vi "dB(T)_2024.vi"(14 "Temperature (K)":dbl=373.15 format="%.4g") -> (0 "T^2*d^2Bair/dT^2":dbl=-9.863442284460733e-05 format="%#_6e", 1 "T*dBair/dT":dbl=4.3077522102604444e-05, 3 "T*dBwater/dT":dbl=0.0016857833537860616 format="%#_6e", 4 "T^2*d^2Bwater/dT^2":dbl=-0.009822685834053062 format="%#_6e", 7 "d^2Bair-water/dT^2":dbl=-1.0645256351379218e-09, 8 "T^2*d^2Bair-water/dT^2":dbl=-0.0001482255314615026 format="%_6e", 9 "dBair-water/dT":dbl=1.5861556674262897e-07, 10 "T*dBair-water/dT":dbl=5.9187398730011994e-05, 11 "dBair/dT":dbl=1.1544291063273333e-07, 12 "d^2Bair/dT^2":dbl=-7.083723741101137e-10, 13 "d^2Bwater/dT^2":dbl=-7.054453286930115e-08, 15 "dBwater/dT":dbl=4.517709644341583e-06)   [LabVIEW 2016]
uses:
  SOS_Global_2022.vi
  <vilib>/gmath/NI_Gmath.lvlib
  <vilib>/Analysis/NI_AALPro.lvlib
panel:
  in  "method interpolation 5":i32(ring)=2 items=["nearest", "linear", "spline", "cubic Hermite", "Lagrange"]
  in  "method derivatives 5":u16(ring)=2 items=["2nd Order Central", "4th Order Central", "Forward", "Backward"]
  in  "method interpolation 4":i32(ring)=2 items=["nearest", "linear", "spline", "cubic Hermite", "Lagrange"]
  in  "method derivatives 4":u16(ring)=2 items=["2nd Order Central", "4th Order Central", "Forward", "Backward"]
  in  "method interpolation 3":i32(ring)=2 items=["nearest", "linear", "spline", "cubic Hermite", "Lagrange"]
  in  "method derivatives 3":u16(ring)=2 items=["2nd Order Central", "4th Order Central", "Forward", "Backward"]
  in  "Bdw source air-water interaction virial":i32(listbox)=3
  in  "Bw source ref water":i32(listbox)=2
  in  "method derivatives 2":u16(ring)=2 items=["2nd Order Central", "4th Order Central", "Forward", "Backward"]
  in  "method interpolation 2":i32(ring)=2 items=["nearest", "linear", "spline", "cubic Hermite", "Lagrange"]
  in  "method derivatives":u16(ring)=2 items=["2nd Order Central", "4th Order Central", "Forward", "Backward"]
  in  "method interpolation":i32(ring)=2 items=["nearest", "linear", "spline", "cubic Hermite", "Lagrange"]
  in  "B source ref dry air":i32(listbox)=1
  # "(m^3 mol^-1)"
  # "(m^3 mol^-1 K^-1)"
  # "(m^3 mol^-1 K^-2)"
  # "(m^3 mol^-1)"
  # "(m^3 mol^-1)"
  # "(m^3 mol^-1 K^-1)"
  # "(m^3 mol^-1)"
  # "(m^3 mol^-1 K^-2)"
  # "(m^3 mol^-1)"
  # "(m^3 mol^-1 K^-1)"
  # "(m^3 mol^-1)"
  # "(m^3 mol^-1 K^-2)"
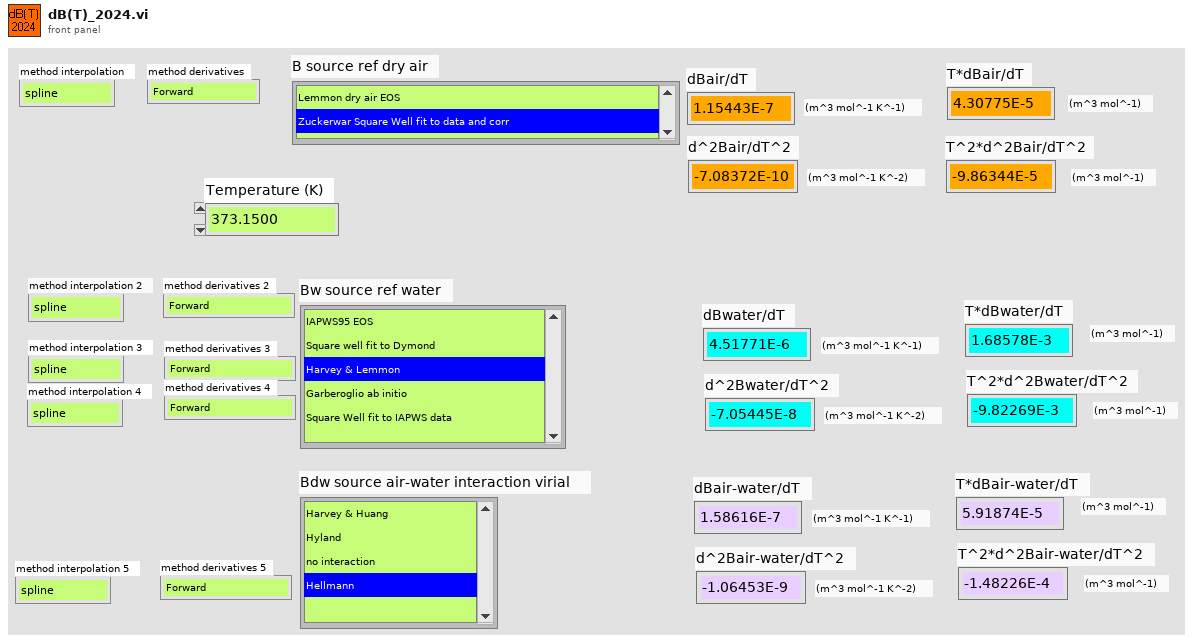
[diagram p1: front panel]
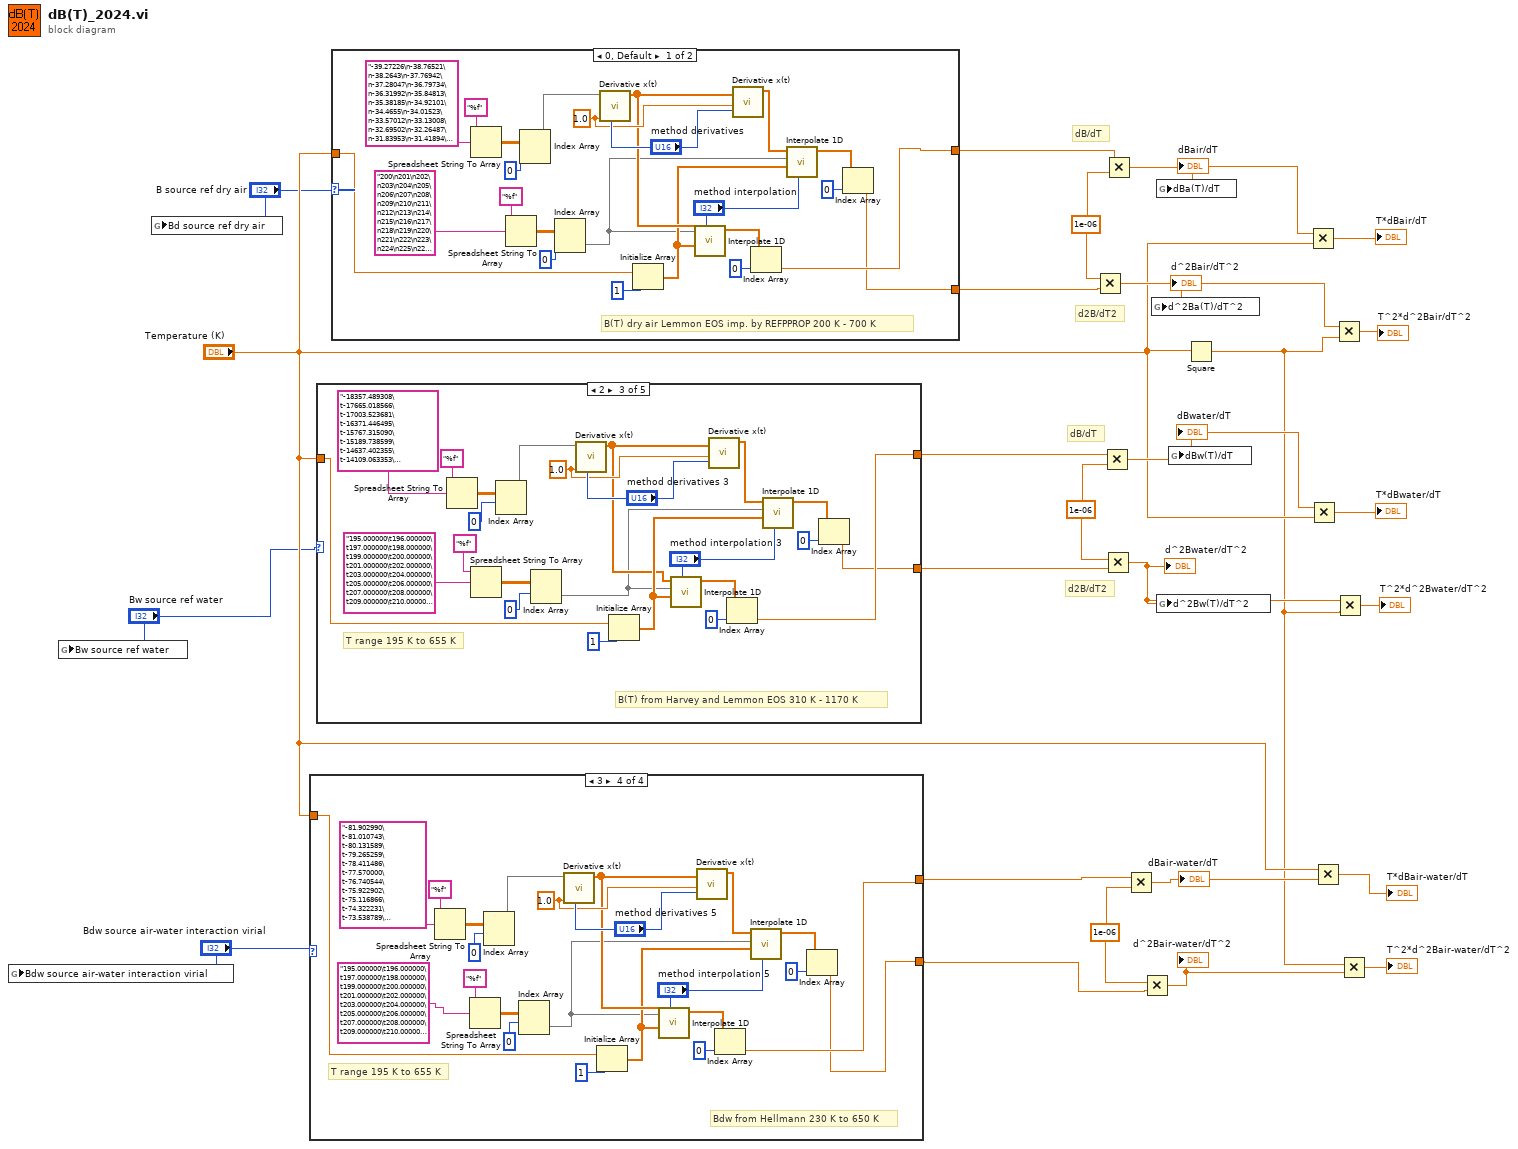
[diagram p0: block diagram]
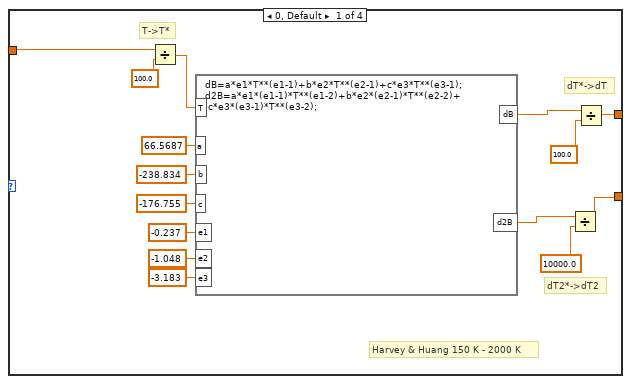
[diagram p2: hidden frame]
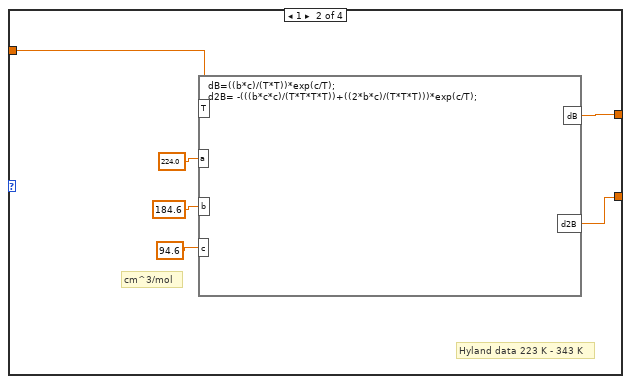
[diagram p3: hidden frame]
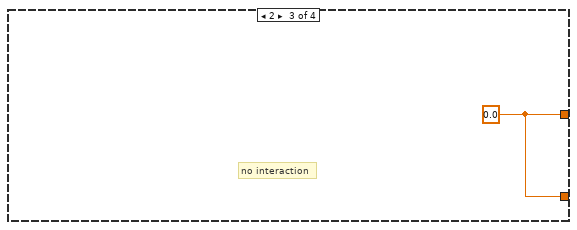
[diagram p4: hidden frame]
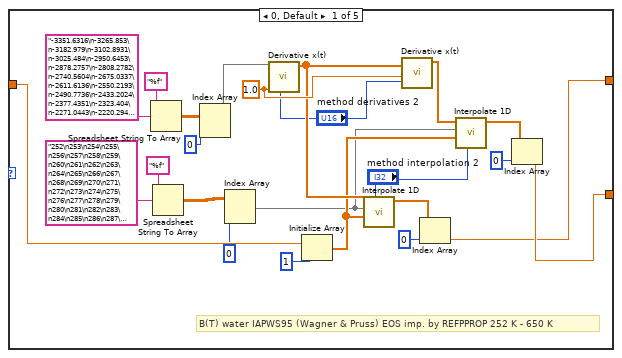
[diagram p5: hidden frame]
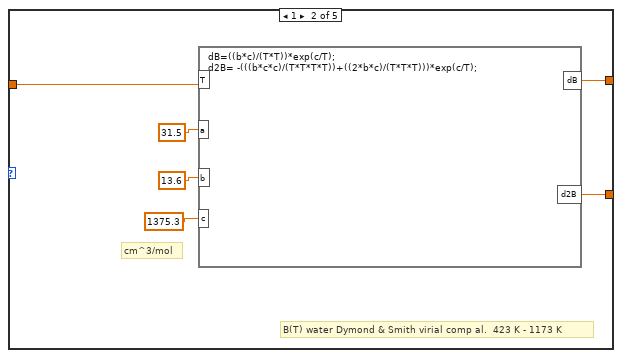
[diagram p6: hidden frame]
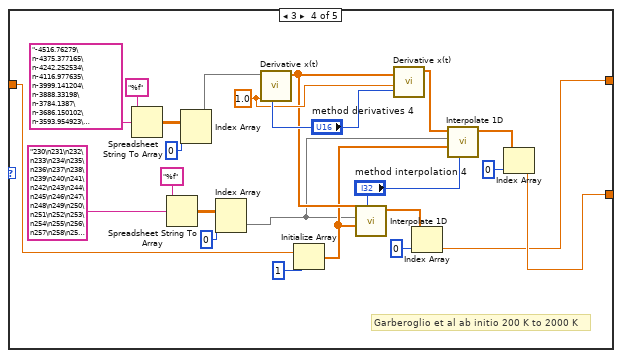
[diagram p7: hidden frame]
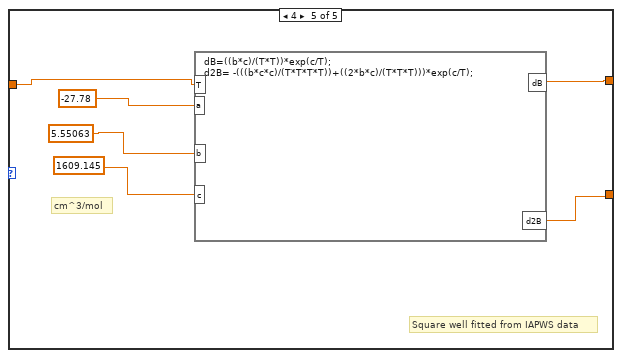
[diagram p8: hidden frame]
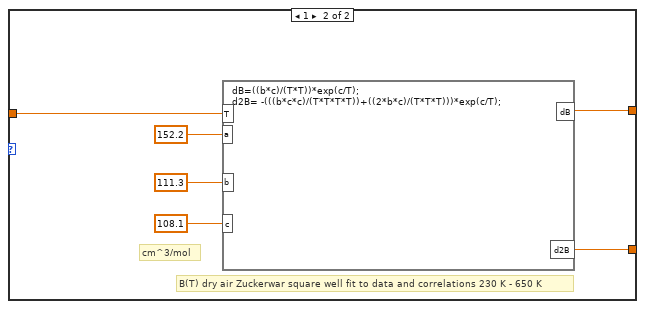
[diagram p9: hidden frame]
diagram:
  w12 = 1e-06 ("y")
  w22 = 1e-06 ("y")
  w23 = 1e-06 ("y")
  # "d2B/dT2"
  # "dB/dT"
  # "d2B/dT2"
  # "dB/dT"
  n1 = global write "SOS_Global_2022.vi" "Bdw source air-water interaction virial"("Bdw source air-water interaction virial") -> ()
  n2 = global write "SOS_Global_2022.vi" "Bw source ref water"("Bw source ref water") -> ()
  n3 = global write "SOS_Global_2022.vi" "Bd source ref dry air"("B source ref dry air") -> ()
  n4 = case shown="3" "Bdw source air-water interaction virial" {
    tunnel: [w31 w44 w48 w55] -> w10
    tunnel: [w30 w43 w48 w54] -> w11
    tunnel: "Temperature (K)" -> [w40 w42 _ w56]
    frame 0, Default {
      # "dT2*->dT2"
      # "dT*->dT"
      # "T->T*"
      # "Harvey & Huang 150 K - 2000 K"
      n5 = Divide(x=w40, y=100.0) -> (x/y=w39:dbl)
      n6 = formula code="dB=a*e1*T**(e1-1)+b*e2*T**(e2-1)+c*e3*T**(e3-1);\nd2B=a*e1*(e1-1)*T**(e1-2)+b*e2*(e2-1)*T**(e2-2)+\n c*e3*(e3-1)*T**(e3-2);"("T"=w39, "a"=66.5687 ("input variable"), "b"=-238.834 ("input variable"), "c"=-176.755 ("input variable"), "e1"=-0.237 ("input variable"), "e2"=-1.048 ("input variable"), "e3"=-3.183 ("input variable")) -> ("dB"=w32:dbl, "d2B"=w28:dbl)
      n7 = Divide(x=w28, y=10000.0) -> (x/y=w30:dbl)
      n8 = Divide(x=w32, y=100.0) -> (x/y=w31:dbl)
    }
    frame 1 {
      # "Hyland data 223 K - 343 K"
      # "cm^3/mol"
      n9 = formula code="dB=((b*c)/(T*T))*exp(c/T);\nd2B= -(((b*c*c)/(T*T*T*T))+((2*b*c)/(T*T*T)))*exp(c/T);"("T"=w42, "a"=224.0 ("input variable"), "b"=184.6 ("input variable"), "c"=94.6 ("input variable")) -> ("dB"=w44:dbl, "d2B"=w43:dbl)
    }
    frame 2 {
      w48 = 0.0
      # "no interaction"
    }
    frame 3 {
      w71 = 1.0 ("dt")
      # "T range 195 K to 655 K"
      # "Bdw from Hellmann 230 K to 650 K"
      n10 = Spreadsheet String To Array(format string="%f", spreadsheet string="-81.902990\t-81.010743\t-80.131589\t-79.265259\t-78.411486\t-77.570000\t-76.740544\t-75.922902\t-75.116866\t-74.322231\t-73.538789\t-72.766335\t-72.004661\t-71.253562\t-70.512830\t-69.782260\t-69.061644\t-68.350777\t-67.649452\t-66.957462\t-66.274601\t-65.600662\t-64.935439\t-64.278725\t-63.630314\t-62.990000\t-62.357591\t-61.732959\t-61.115989\t-60.506569\t-59.904585\t-59.309924\t-58.722471\t-58.142115\t-57.568740\t-57.002235\t-56.442484\t-55.889376\t-55.342796\t-54.802631\t-54.268767\t-53.741092\t-53.219491\t-52.703851\t-52.194058\t-51.690000\t-51.191569\t-50.698684\t-50.211270\t-49.729254\t-49.252559\t-48.781111\t-48.314836\t-47.853660\t-47.397506\t-46.946301\t-46.499970\t-46.058439\t-45.621632\t-45.189475\t-44.761893\t-44.338812\t-43.920157\t-43.505853\t-43.095825\t-42.690000\t-42.288305\t-41.890685\t-41.497087\t-41.107457\t-40.721743\t-40.339892\t-39.961851\t-39.587567\t-39.216988\t-38.850061\t-38.486732\t-38.126949\t-37.770660\t-37.417810\t-37.068348\t-36.722221\t-36.379375\t-36.039758\t-35.703318\t-35.370000\t-35.039755\t-34.712545\t-34.388332\t-34.067080\t-33.748752\t-33.433312\t-33.120725\t-32.810952\t-32.503958\t-32.199707\t-31.898161\t-31.599285\t-31.303041\t-31.009395\t-30.718308\t-30.429745\t-30.143669\t-29.860044\t-29.578833\t-29.300000\t-29.023511\t-28.749343\t-28.477474\t-28.207884\t-27.940552\t-27.675458\t-27.412580\t-27.151897\t-26.893390\t-26.637036\t-26.382815\t-26.130707\t-25.880690\t-25.632744\t-25.386847\t-25.142980\t-24.901120\t-24.661248\t-24.423343\t-24.187383\t-23.953347\t-23.721216\t-23.490968\t-23.262583\t-23.036038\t-22.811315\t-22.588391\t-22.367247\t-22.147860\t-21.930211\t-21.714279\t-21.500042\t-21.287480\t-21.076572\t-20.867297\t-20.659635\t-20.453564\t-20.249064\t-20.046114\t-19.844693\t-19.644780\t-19.446355\t-19.249396\t-19.053883\t-18.859795\t-18.667111\t-18.475811\t-18.285872\t-18.097276\t-17.910000\t-17.724026\t-17.539342\t-17.355939\t-17.173806\t-16.992934\t-16.813313\t-16.634933\t-16.457785\t-16.281858\t-16.107144\t-15.933631\t-15.761311\t-15.590173\t-15.420208\t-15.251406\t-15.083758\t-14.917252\t-14.751881\t-14.587633\t-14.424499\t-14.262470\t-14.101535\t-13.941685\t-13.782909\t-13.625199\t-13.468544\t-13.312935\t-13.158362\t-13.004814\t-12.852283\t-12.700758\t-12.550230\t-12.400689\t-12.252125\t-12.104528\t-11.957889\t-11.812197\t-11.667444\t-11.523618\t-11.380711\t-11.238713\t-11.097613\t-10.957403\t-10.818072\t-10.679610\t-10.542007\t-10.405255\t-10.269343\t-10.134261\t-10.000000\t-9.866550\t-9.733906\t-9.602062\t-9.471012\t-9.340753\t-9.211277\t-9.082580\t-8.954657\t-8.827502\t-8.701110\t-8.575475\t-8.450593\t-8.326458\t-8.203064\t-8.080407\t-7.958481\t-7.837281\t-7.716800\t-7.597036\t-7.477980\t-7.359630\t-7.241978\t-7.125020\t-7.008751\t-6.893165\t-6.778257\t-6.664021\t-6.550452\t-6.437546\t-6.325296\t-6.213697\t-6.102745\t-5.992433\t-5.882756\t-5.773710\t-5.665288\t-5.557485\t-5.450297\t-5.343717\t-5.237741\t-5.132363\t-5.027578\t-4.923380\t-4.819765\t-4.716726\t-4.614259\t-4.512358\t-4.411018\t-4.310234\t-4.210000\t-4.110311\t-4.011164\t-3.912555\t-3.814480\t-3.716936\t-3.619920\t-3.523427\t-3.427455\t-3.331999\t-3.237057\t-3.142625\t-3.048699\t-2.955276\t-2.862353\t-2.769925\t-2.677989\t-2.586542\t-2.495581\t-2.405101\t-2.315099\t-2.225573\t-2.136517\t-2.047929\t-1.959805\t-1.872142\t-1.784936\t-1.698183\t-1.611881\t-1.526025\t-1.440613\t-1.355640\t-1.271103\t-1.186999\t-1.103323\t-1.020073\t-0.937246\t-0.854836\t-0.772842\t-0.691259\t-0.610084\t-0.529314\t-0.448944\t-0.368972\t-0.289394\t-0.210206\t-0.131405\t-0.052988\t0.025050\t0.102711\t0.180000\t0.256919\t0.333470\t0.409656\t0.485478\t0.560938\t0.636038\t0.710780\t0.785165\t0.859196\t0.932874\t1.006201\t1.079178\t1.151809\t1.224094\t1.296036\t1.367635\t1.438895\t1.509817\t1.580403\t1.650654\t1.720572\t1.790160\t1.859419\t1.928351\t1.996958\t2.065241\t2.133203\t2.200845\t2.268169\t2.335177\t2.401871\t2.468253\t2.534324\t2.600086\t2.665542\t2.730693\t2.795540\t2.860086\t2.924333\t2.988282\t3.051935\t3.115294\t3.178361\t3.241138\t3.303626\t3.365828\t3.427744\t3.489378\t3.550731\t3.611804\t3.672600\t3.733121\t3.793367\t3.853342\t3.913047\t3.972483\t4.031653\t4.090558\t4.149201\t4.207583\t4.265705\t4.323571\t4.381181\t4.438537\t4.495642\t4.552497\t4.609104\t4.665464\t4.721581\t4.777454\t4.833087\t4.888481\t4.943638\t4.998560\t5.053249\t5.107706\t5.161933\t5.215933\t5.269707\t5.323256\t5.376583\t5.429690\t5.482578\t5.535249\t5.587705\t5.639948\t5.691980\t5.743802\t5.795417\t5.846825\t5.898030\t5.949033\t5.999836\t6.050440\t6.100847\t6.151060\t6.201080\t6.250908\t6.300548\t6.350000\t6.399266\t6.448348\t6.497244\t6.545957\t6.594487\t6.642834\t6.690999\t6.738983\t6.786786\t6.834408\t6.881851\t6.929114\t6.976199\t7.023106\t7.069836\t7.116389\t7.162765\t7.208966\t7.254992\t7.300844\t7.346521\t7.392025\t7.437357\t7.482516\t7.527504\t7.572321\t7.616968\t7.661445\t7.705752\t7.749891\t7.793862\t7.837665\t7.881302\t7.924772\t7.968077\t8.011217\t8.054192\t8.097003\t8.139650\t8.182135\t8.224458\t8.266619\t8.308619\t8.350459\t8.392139\t8.433660\t8.475021\t8.516225\t8.557272\t8.598161\t8.638894\t8.679471\t8.719894\t8.760161\t8.800275" ("B dw Hellmann array")) -> (array=w58:dbl[][])  [unwired: 2 in]
      n11 = Spreadsheet String To Array(format string="%f", spreadsheet string="195.000000\t196.000000\t197.000000\t198.000000\t199.000000\t200.000000\t201.000000\t202.000000\t203.000000\t204.000000\t205.000000\t206.000000\t207.000000\t208.000000\t209.000000\t210.000000\t211.000000\t212.000000\t213.000000\t214.000000\t215.000000\t216.000000\t217.000000\t218.000000\t219.000000\t220.000000\t221.000000\t222.000000\t223.000000\t224.000000\t225.000000\t226.000000\t227.000000\t228.000000\t229.000000\t230.000000\t231.000000\t232.000000\t233.000000\t234.000000\t235.000000\t236.000000\t237.000000\t238.000000\t239.000000\t240.000000\t241.000000\t242.000000\t243.000000\t244.000000\t245.000000\t246.000000\t247.000000\t248.000000\t249.000000\t250.000000\t251.000000\t252.000000\t253.000000\t254.000000\t255.000000\t256.000000\t257.000000\t258.000000\t259.000000\t260.000000\t261.000000\t262.000000\t263.000000\t264.000000\t265.000000\t266.000000\t267.000000\t268.000000\t269.000000\t270.000000\t271.000000\t272.000000\t273.000000\t274.000000\t275.000000\t276.000000\t277.000000\t278.000000\t279.000000\t280.000000\t281.000000\t282.000000\t283.000000\t284.000000\t285.000000\t286.000000\t287.000000\t288.000000\t289.000000\t290.000000\t291.000000\t292.000000\t293.000000\t294.000000\t295.000000\t296.000000\t297.000000\t298.000000\t299.000000\t300.000000\t301.000000\t302.000000\t303.000000\t304.000000\t305.000000\t306.000000\t307.000000\t308.000000\t309.000000\t310.000000\t311.000000\t312.000000\t313.000000\t314.000000\t315.000000\t316.000000\t317.000000\t318.000000\t319.000000\t320.000000\t321.000000\t322.000000\t323.000000\t324.000000\t325.000000\t326.000000\t327.000000\t328.000000\t329.000000\t330.000000\t331.000000\t332.000000\t333.000000\t334.000000\t335.000000\t336.000000\t337.000000\t338.000000\t339.000000\t340.000000\t341.000000\t342.000000\t343.000000\t344.000000\t345.000000\t346.000000\t347.000000\t348.000000\t349.000000\t350.000000\t351.000000\t352.000000\t353.000000\t354.000000\t355.000000\t356.000000\t357.000000\t358.000000\t359.000000\t360.000000\t361.000000\t362.000000\t363.000000\t364.000000\t365.000000\t366.000000\t367.000000\t368.000000\t369.000000\t370.000000\t371.000000\t372.000000\t373.000000\t374.000000\t375.000000\t376.000000\t377.000000\t378.000000\t379.000000\t380.000000\t381.000000\t382.000000\t383.000000\t384.000000\t385.000000\t386.000000\t387.000000\t388.000000\t389.000000\t390.000000\t391.000000\t392.000000\t393.000000\t394.000000\t395.000000\t396.000000\t397.000000\t398.000000\t399.000000\t400.000000\t401.000000\t402.000000\t403.000000\t404.000000\t405.000000\t406.000000\t407.000000\t408.000000\t409.000000\t410.000000\t411.000000\t412.000000\t413.000000\t414.000000\t415.000000\t416.000000\t417.000000\t418.000000\t419.000000\t420.000000\t421.000000\t422.000000\t423.000000\t424.000000\t425.000000\t426.000000\t427.000000\t428.000000\t429.000000\t430.000000\t431.000000\t432.000000\t433.000000\t434.000000\t435.000000\t436.000000\t437.000000\t438.000000\t439.000000\t440.000000\t441.000000\t442.000000\t443.000000\t444.000000\t445.000000\t446.000000\t447.000000\t448.000000\t449.000000\t450.000000\t451.000000\t452.000000\t453.000000\t454.000000\t455.000000\t456.000000\t457.000000\t458.000000\t459.000000\t460.000000\t461.000000\t462.000000\t463.000000\t464.000000\t465.000000\t466.000000\t467.000000\t468.000000\t469.000000\t470.000000\t471.000000\t472.000000\t473.000000\t474.000000\t475.000000\t476.000000\t477.000000\t478.000000\t479.000000\t480.000000\t481.000000\t482.000000\t483.000000\t484.000000\t485.000000\t486.000000\t487.000000\t488.000000\t489.000000\t490.000000\t491.000000\t492.000000\t493.000000\t494.000000\t495.000000\t496.000000\t497.000000\t498.000000\t499.000000\t500.000000\t501.000000\t502.000000\t503.000000\t504.000000\t505.000000\t506.000000\t507.000000\t508.000000\t509.000000\t510.000000\t511.000000\t512.000000\t513.000000\t514.000000\t515.000000\t516.000000\t517.000000\t518.000000\t519.000000\t520.000000\t521.000000\t522.000000\t523.000000\t524.000000\t525.000000\t526.000000\t527.000000\t528.000000\t529.000000\t530.000000\t531.000000\t532.000000\t533.000000\t534.000000\t535.000000\t536.000000\t537.000000\t538.000000\t539.000000\t540.000000\t541.000000\t542.000000\t543.000000\t544.000000\t545.000000\t546.000000\t547.000000\t548.000000\t549.000000\t550.000000\t551.000000\t552.000000\t553.000000\t554.000000\t555.000000\t556.000000\t557.000000\t558.000000\t559.000000\t560.000000\t561.000000\t562.000000\t563.000000\t564.000000\t565.000000\t566.000000\t567.000000\t568.000000\t569.000000\t570.000000\t571.000000\t572.000000\t573.000000\t574.000000\t575.000000\t576.000000\t577.000000\t578.000000\t579.000000\t580.000000\t581.000000\t582.000000\t583.000000\t584.000000\t585.000000\t586.000000\t587.000000\t588.000000\t589.000000\t590.000000\t591.000000\t592.000000\t593.000000\t594.000000\t595.000000\t596.000000\t597.000000\t598.000000\t599.000000\t600.000000\t601.000000\t602.000000\t603.000000\t604.000000\t605.000000\t606.000000\t607.000000\t608.000000\t609.000000\t610.000000\t611.000000\t612.000000\t613.000000\t614.000000\t615.000000\t616.000000\t617.000000\t618.000000\t619.000000\t620.000000\t621.000000\t622.000000\t623.000000\t624.000000\t625.000000\t626.000000\t627.000000\t628.000000\t629.000000\t630.000000\t631.000000\t632.000000\t633.000000\t634.000000\t635.000000\t636.000000\t637.000000\t638.000000\t639.000000\t640.000000\t641.000000\t642.000000\t643.000000\t644.000000\t645.000000\t646.000000\t647.000000\t648.000000\t649.000000\t650.000000\t651.000000\t652.000000\t653.000000\t654.000000\t655.000000" ("string T array")) -> (array=w60:dbl[][])  [unwired: 2 in]
      n12 = Index Array(array=w58, index (row)=0 ("disabled index (col)")) -> (element=w57:dbl[])  [unwired: 1 in]
      n13 = Index Array(array=w60, index (row)=0 ("disabled index (col)")) -> (element=w53:dbl[])  [unwired: 1 in]
      n14 = call <vilib>:"Derivative x(t).vi"("method"="method derivatives 5", "dt"=w71, "X"=w57) -> ("dX/dt"=w64:dbl[])  [unwired: 7 in, 1 out]
      n15 = Initialize Array(w56, 1 ("dimension size")) -> (w63:dbl[])
      n16 = call <vilib>:"Interpolate 1D.vi"("method"="method interpolation 5", "xi"=w63, "X"=w53, "Y"=w64) -> ("yi"=w69:dbl[])  [unwired: 5 in, 2 out]
      n17 = call <vilib>:"Derivative x(t).vi"("method"="method derivatives 5", "dt"=w71, "X"=w64) -> ("dX/dt"=w65:dbl[])  [unwired: 7 in, 1 out]
      n18 = Index Array(array=w69, index=0) -> (element=w55:dbl)
      n19 = call <vilib>:"Interpolate 1D.vi"("method"="method interpolation 5", "xi"=w63, "X"=w53, "Y"=w65) -> ("yi"=w67:dbl[])  [unwired: 5 in, 2 out]
      n20 = Index Array(array=w67, index=0) -> (element=w54:dbl)
    }
  }
  n21 = case shown="2" "Bw source ref water" {
    tunnel: [w85 w99 w111 w129 w153] -> w25
    tunnel: [w86 w98 w110 w130 w152] -> w21
    tunnel: "Temperature (K)" -> [w83 w97 w112 w131 w151]
    frame 0, Default {
      w96 = 1.0 ("dt")
      # "B(T) water IAPWS95 (Wagner & Pruss) EOS imp. by REFPPROP 252 K - 650 K"
      n22 = Spreadsheet String To Array(format string="%f", spreadsheet string="-3351.6316\n-3265.853\n-3182.979\n-3102.8931\n-3025.484\n-2950.6453\n-2878.2757\n-2808.2782\n-2740.5604\n-2675.0337\n-2611.6136\n-2550.2193\n-2490.7736\n-2433.2024\n-2377.4351\n-2323.404\n-2271.0443\n-2220.294\n-2171.0936\n-2123.3865\n-2077.1179\n-2032.2357\n-1988.6898\n-1946.4323\n-1905.4172\n-1865.6002\n-1826.9391\n-1789.3932\n-1752.9236\n-1717.4929\n-1683.065\n-1649.6055\n-1617.0813\n-1585.4606\n-1554.7126\n-1524.8081\n-1495.7188\n-1467.4174\n-1439.8779\n-1413.0752\n-1386.985\n-1361.5841\n-1336.8502\n-1312.7616\n-1289.2976\n-1266.4383\n-1244.1643\n-1222.4573\n-1201.2993\n-1180.6731\n-1160.5622\n-1140.9505\n-1121.8228\n-1103.164\n-1084.96\n-1067.1968\n-1049.8612\n-1032.9402\n-1016.4216\n-1000.2932\n-984.54359\n-969.16154\n-954.13627\n-939.45738\n-925.1148\n-911.09882\n-897.40004\n-884.0094\n-870.91812\n-858.11771\n-845.59999\n-833.35702\n-821.38114\n-809.66492\n-798.2012\n-786.98303\n-776.0037\n-765.25669\n-754.73573\n-744.43471\n-734.34773\n-724.46907\n-714.79322\n-705.3148\n-696.02862\n-686.92965\n-678.01302\n-669.27399\n-660.70798\n-652.31057\n-644.07743\n-636.00439\n-628.08741\n-620.32255\n-612.706\n-605.23407\n-597.90317\n-590.70981\n-583.65063\n-576.72233\n-569.92173\n-563.24575\n-556.69137\n-550.25568\n-543.93585\n-537.72913\n-531.63285\n-525.6444\n-519.76126\n-513.98098\n-508.30118\n-502.71953\n-497.23378\n-491.84174\n-486.54128\n-481.33032\n-476.20686\n-471.16892\n-466.2146\n-461.34205\n-456.54945\n-451.83504\n-447.19713\n-442.63403\n-438.14413\n-433.72584\n-429.37763\n-425.09801\n-420.8855\n-416.7387\n-412.65621\n-408.63669\n-404.67882\n-400.78132\n-396.94294\n-393.16247\n-389.43872\n-385.77053\n-382.15678\n-378.59636\n-375.08821\n-371.63127\n-368.22453\n-364.86699\n-361.55769\n-358.29567\n-355.08\n-351.9098\n-348.78417\n-345.70225\n-342.66322\n-339.66625\n-336.71053\n-333.7953\n-330.91978\n-328.08323\n-325.28492\n-322.52415\n-319.80022\n-317.11245\n-314.46018\n-311.84275\n-309.25955\n-306.70994\n-304.19333\n-301.70912\n-299.25674\n-296.83561\n-294.4452\n-292.08495\n-289.75434\n-287.45285\n-285.17998\n-282.93524\n-280.71813\n-278.52818\n-276.36494\n-274.22795\n-272.11676\n-270.03094\n-267.97007\n-265.93373\n-263.92151\n-261.93301\n-259.96785\n-258.02564\n-256.106\n-254.20858\n-252.333\n-250.47892\n-248.646\n-246.8339\n-245.04228\n-243.27082\n-241.5192\n-239.78712\n-238.07426\n-236.38033\n-234.70504\n-233.04809\n-231.40921\n-229.78812\n-228.18454\n-226.59822\n-225.02889\n-223.4763\n-221.94019\n-220.42032\n-218.91645\n-217.42834\n-215.95576\n-214.49849\n-213.05629\n-211.62895\n-210.21626\n-208.81799\n-207.43396\n-206.06394\n-204.70775\n-203.36518\n-202.03604\n-200.72015\n-199.41732\n-198.12736\n-196.8501\n-195.58536\n-194.33297\n-193.09275\n-191.86455\n-190.64819\n-189.44352\n-188.25038\n-187.06861\n-185.89806\n-184.73858\n-183.59003\n-182.45225\n-181.3251\n-180.20846\n-179.10217\n-178.0061\n-176.92012\n-175.8441\n-174.77791\n-173.72142\n-172.67451\n-171.63706\n-170.60894\n-169.59004\n-168.58024\n-167.57943\n-166.58749\n-165.60432\n-164.6298\n-163.66382\n-162.70629\n-161.75709\n-160.81613\n-159.88331\n-158.95852\n-158.04167\n-157.13265\n-156.23139\n-155.33778\n-154.45174\n-153.57316\n-152.70198\n-151.83808\n-150.9814\n-150.13185\n-149.28933\n-148.45378\n-147.62511\n-146.80324\n-145.98809\n-145.17958\n-144.37764\n-143.58219\n-142.79316\n-142.01048\n-141.23407\n-140.46386\n-139.69979\n-138.94179\n-138.18978\n-137.4437\n-136.70348\n-135.96907\n-135.24039\n-134.51739\n-133.79999\n-133.08815\n-132.3818\n-131.68087\n-130.98532\n-130.29508\n-129.6101\n-128.93032\n-128.25568\n-127.58614\n-126.92163\n-126.2621\n-125.6075\n-124.95779\n-124.3129\n-123.67279\n-123.03741\n-122.4067\n-121.78063\n-121.15914\n-120.54219\n-119.92972\n-119.3217\n-118.71808\n-118.11881\n-117.52386\n-116.93317\n-116.3467\n-115.76441\n-115.18627\n-114.61222\n-114.04223\n-113.47625\n-112.91426\n-112.3562\n-111.80204\n-111.25175\n-110.70528\n-110.16259\n-109.62366\n-109.08844\n-108.5569\n-108.029\n-107.50471\n-106.98399\n-106.46682\n-105.95314\n-105.44294\n-104.93618\n-104.43283\n-103.93285\n-103.43622\n-102.9429\n-102.45286\n-101.96607\n-101.4825\n-101.00212\n-100.5249\n-100.05082\n-99.57984\n-99.11194\n-98.64708\n-98.18524\n-97.72639\n-97.27052\n-96.81757\n-96.36755\n-95.9204\n-95.47612\n-95.03467\n-94.59603\n-94.16017\n-93.72708\n-93.29672\n-92.86907\n-92.44411\n-92.02181\n-91.60216\n-91.18512\n-90.77067\n-90.3588\n-89.94948\n-89.54269\n-89.1384\n-88.73659\n-88.33726\n-87.94036\n-87.54588\n-87.15381\n-86.76412\n-86.37678\n-85.99179\n-85.60912\n-85.22875\n-84.85067\n-84.47484\n-84.10126\n-83.72991\n-83.36076\n-82.9938\n-82.62901\n-82.26638\n-81.90588\n-81.5475\n-81.19122\n-80.83702\n-80.48489\n-80.13481\n-79.78676") -> (array=w78:dbl[][])  [unwired: 2 in]
      n23 = Spreadsheet String To Array(format string="%f", spreadsheet string="252\n253\n254\n255\n256\n257\n258\n259\n260\n261\n262\n263\n264\n265\n266\n267\n268\n269\n270\n271\n272\n273\n274\n275\n276\n277\n278\n279\n280\n281\n282\n283\n284\n285\n286\n287\n288\n289\n290\n291\n292\n293\n294\n295\n296\n297\n298\n299\n300\n301\n302\n303\n304\n305\n306\n307\n308\n309\n310\n311\n312\n313\n314\n315\n316\n317\n318\n319\n320\n321\n322\n323\n324\n325\n326\n327\n328\n329\n330\n331\n332\n333\n334\n335\n336\n337\n338\n339\n340\n341\n342\n343\n344\n345\n346\n347\n348\n349\n350\n351\n352\n353\n354\n355\n356\n357\n358\n359\n360\n361\n362\n363\n364\n365\n366\n367\n368\n369\n370\n371\n372\n373\n374\n375\n376\n377\n378\n379\n380\n381\n382\n383\n384\n385\n386\n387\n388\n389\n390\n391\n392\n393\n394\n395\n396\n397\n398\n399\n400\n401\n...") -> (array=w81:dbl[][])  [unwired: 2 in]
      n24 = Index Array(array=w78, index (col)=0 ("disabled index (col)")) -> (element=w74:dbl[])  [unwired: 1 in]
      n25 = Index Array(array=w81, index (col)=0 ("disabled index (col)")) -> (element=w73:dbl[])  [unwired: 1 in]
      n26 = call <vilib>:"Derivative x(t).vi"("method"="method derivatives 2", "dt"=w96, "X"=w74) -> ("dX/dt"=w89:dbl[])  [unwired: 7 in, 1 out]
      n27 = Initialize Array(w83, 1 ("dimension size")) -> (w88:dbl[])
      n28 = call <vilib>:"Interpolate 1D.vi"("method"="method interpolation 2", "xi"=w88, "X"=w73, "Y"=w89) -> ("yi"=w94:dbl[])  [unwired: 5 in, 2 out]
      n29 = call <vilib>:"Derivative x(t).vi"("method"="method derivatives 2", "dt"=w96, "X"=w89) -> ("dX/dt"=w90:dbl[])  [unwired: 7 in, 1 out]
      n30 = Index Array(array=w94, index=0) -> (element=w85:dbl)
      n31 = call <vilib>:"Interpolate 1D.vi"("method"="method interpolation 2", "xi"=w88, "X"=w73, "Y"=w90) -> ("yi"=w92:dbl[])  [unwired: 5 in, 2 out]
      n32 = Index Array(array=w92, index=0) -> (element=w86:dbl)
    }
    frame 1 {
      # "B(T) water Dymond & Smith virial comp al.  423 K - 1173 K"
      # "cm^3/mol"
      n33 = formula code="dB=((b*c)/(T*T))*exp(c/T);\nd2B= -(((b*c*c)/(T*T*T*T))+((2*b*c)/(T*T*T)))*exp(c/T);"("T"=w97, "a"=31.5 ("input variable"), "b"=13.6 ("input variable"), "c"=1375.3 ("input variable")) -> ("dB"=w99:dbl, "d2B"=w98:dbl)
    }
    frame 2 {
      w125 = 1.0 ("dt")
      # "T range 195 K to 655 K"
      # "B(T) from Harvey and Lemmon EOS 310 K - 1170 K"
      n34 = Spreadsheet String To Array(format string="%f", spreadsheet string="-18357.489308\t-17665.018566\t-17003.523681\t-16371.446495\t-15767.315090\t-15189.738599\t-14637.402355\t-14109.063353\t-13603.546005\t-13119.738158\t-12656.587379\t-12213.097459\t-11788.325153\t-11381.377113\t-10991.407015\t-10617.612868\t-10259.234487\t-9915.551116\t-9585.879208\t-9269.570329\t-8966.009198\t-8674.611835\t-8394.823834\t-8126.118725\t-7867.996445\t-7619.981892\t-7381.623567\t-7152.492297\t-6932.180032\t-6720.298710\t-6516.479192\t-6320.370249\t-6131.637624\t-5949.963127\t-5775.043802\t-5606.591122\t-5444.330246\t-5287.999305\t-5137.348738\t-4992.140656\t-4852.148249\t-4717.155220\t-4586.955255\t-4461.351516\t-4340.156169\t-4223.189931\t-4110.281646\t-4001.267879\t-3895.992540\t-3794.306519\t-3696.067345\t-3601.138863\t-3509.390928\t-3420.699114\t-3334.944438\t-3252.013100\t-3171.796234\t-3094.189677\t-3019.093744\t-2946.413014\t-2876.056137\t-2807.935638\t-2741.967737\t-2678.072179\t-2616.172074\t-2556.193734\t-2498.066536\t-2441.722776\t-2387.097538\t-2334.128567\t-2282.756150\t-2232.923004\t-2184.574163\t-2137.656875\t-2092.120510\t-2047.916459\t-2004.998048\t-1963.320453\t-1922.840620\t-1883.517186\t-1845.310409\t-1808.182094\t-1772.095528\t-1737.015420\t-1702.907834\t-1669.740137\t-1637.480939\t-1606.100048\t-1575.568409\t-1545.858066\t-1516.942111\t-1488.794643\t-1461.390724\t-1434.706342\t-1408.718370\t-1383.404533\t-1358.743371\t-1334.714205\t-1311.297109\t-1288.472878\t-1266.222998\t-1244.529617\t-1223.375525\t-1202.744121\t-1182.619393\t-1162.985895\t-1143.828722\t-1125.133492\t-1106.886324\t-1089.073819\t-1071.683041\t-1054.701499\t-1038.117131\t-1021.918286\t-1006.093710\t-990.632529\t-975.524239\t-960.758685\t-946.326053\t-932.216857\t-918.421926\t-904.932389\t-891.739672\t-878.835477\t-866.211781\t-853.860819\t-841.775079\t-829.947291\t-818.370418\t-807.037649\t-795.942389\t-785.078253\t-774.439057\t-764.018813\t-753.811719\t-743.812156\t-734.014677\t-724.414007\t-715.005031\t-705.782793\t-696.742486\t-687.879453\t-679.189176\t-670.667273\t-662.309496\t-654.111722\t-646.069953\t-638.180309\t-630.439025\t-622.842447\t-615.387028\t-608.069325\t-600.885996\t-593.833795\t-586.909569\t-580.110259\t-573.432890\t-566.874573\t-560.432503\t-554.103952\t-547.886270\t-541.776881\t-535.773283\t-529.873040\t-524.073786\t-518.373221\t-512.769106\t-507.259266\t-501.841583\t-496.513997\t-491.274506\t-486.121160\t-481.052060\t-476.065361\t-471.159265\t-466.332023\t-461.581931\t-456.907330\t-452.306605\t-447.778183\t-443.320532\t-438.932159\t-434.611611\t-430.357470\t-426.168357\t-422.042925\t-417.979864\t-413.977896\t-410.035774\t-406.152284\t-402.326242\t-398.556492\t-394.841909\t-391.181393\t-387.573874\t-384.018305\t-380.513667\t-377.058965\t-373.653227\t-370.295505\t-366.984875\t-363.720433\t-360.501299\t-357.326610\t-354.195527\t-351.107230\t-348.060916\t-345.055803\t-342.091126\t-339.166139\t-336.280111\t-333.432330\t-330.622098\t-327.848735\t-325.111575\t-322.409968\t-319.743277\t-317.110882\t-314.512174\t-311.946559\t-309.413456\t-306.912296\t-304.442524\t-302.003595\t-299.594978\t-297.216152\t-294.866608\t-292.545848\t-290.253384\t-287.988739\t-285.751446\t-283.541048\t-281.357096\t-279.199154\t-277.066792\t-274.959589\t-272.877135\t-270.819026\t-268.784869\t-266.774276\t-264.786869\t-262.822277\t-260.880137\t-258.960093\t-257.061795\t-255.184901\t-253.329078\t-251.493995\t-249.679332\t-247.884772\t-246.110007\t-244.354732\t-242.618650\t-240.901471\t-239.202906\t-237.522677\t-235.860508\t-234.216128\t-232.589274\t-230.979685\t-229.387107\t-227.811289\t-226.251986\t-224.708957\t-223.181967\t-221.670782\t-220.175176\t-218.694925\t-217.229809\t-215.779614\t-214.344127\t-212.923141\t-211.516452\t-210.123860\t-208.745168\t-207.380184\t-206.028717\t-204.690581\t-203.365593\t-202.053573\t-200.754345\t-199.467734\t-198.193571\t-196.931687\t-195.681919\t-194.444103\t-193.218081\t-192.003697\t-190.800796\t-189.609227\t-188.428843\t-187.259496\t-186.101043\t-184.953343\t-183.816257\t-182.689648\t-181.573382\t-180.467327\t-179.371352\t-178.285331\t-177.209136\t-176.142645\t-175.085735\t-174.038287\t-173.000184\t-171.971308\t-170.951546\t-169.940786\t-168.938916\t-167.945829\t-166.961417\t-165.985575\t-165.018199\t-164.059187\t-163.108438\t-162.165853\t-161.231335\t-160.304788\t-159.386117\t-158.475229\t-157.572033\t-156.676438\t-155.788356\t-154.907698\t-154.034378\t-153.168312\t-152.309416\t-151.457607\t-150.612804\t-149.774927\t-148.943897\t-148.119637\t-147.302069\t-146.491118\t-145.686710\t-144.888772\t-144.097231\t-143.312016\t-142.533057\t-141.760284\t-140.993630\t-140.233027\t-139.478409\t-138.729711\t-137.986867\t-137.249815\t-136.518492\t-135.792836\t-135.072786\t-134.358281\t-133.649264\t-132.945675\t-132.247456\t-131.554551\t-130.866903\t-130.184458\t-129.507161\t-128.834957\t-128.167794\t-127.505620\t-126.848381\t-126.196029\t-125.548511\t-124.905779\t-124.267784\t-123.634476\t-123.005809\t-122.381735\t-121.762207\t-121.147180\t-120.536609\t-119.930448\t-119.328654\t-118.731183\t-118.137991\t-117.549037\t-116.964278\t-116.383674\t-115.807183\t-115.234764\t-114.666378\t-114.101986\t-113.541549\t-112.985027\t-112.432385\t-111.883583\t-111.338585\t-110.797355\t-110.259856\t-109.726052\t-109.195910\t-108.669393\t-108.146467\t-107.627099\t-107.111255\t-106.598902\t-106.090008\t-105.584539\t-105.082464\t-104.583751\t-104.088370\t-103.596289\t-103.107478\t-102.621907\t-102.139546\t-101.660365\t-101.184337\t-100.711431\t-100.241621\t-99.774877\t-99.311171\t-98.850478\t-98.392768\t-97.938017\t-97.486197\t-97.037282\t-96.591246\t-96.148063\t-95.707709\t-95.270159\t-94.835387\t-94.403370\t-93.974083\t-93.547502\t-93.123603\t-92.702364\t-92.283761\t-91.867772\t-91.454373\t-91.043543\t-90.635259\t-90.229499\t-89.826243\t-89.425468\t-89.027153\t-88.631278\t-88.237822\t-87.846764\t-87.458084\t-87.071762\t-86.687779\t-86.306114\t-85.926749\t-85.549663\t-85.174839\t-84.802258\t-84.431900\t-84.063748\t-83.697782\t-83.333987\t-82.972342\t-82.612832\t-82.255438\t-81.900143\t-81.546930\t-81.195782\t-80.846683\t-80.499616\t-80.154565\t-79.811513\t-79.470444" ("B HL array")) -> (array=w114:dbl[][])  [unwired: 2 in]
      n35 = Spreadsheet String To Array(format string="%f", spreadsheet string="195.000000\t196.000000\t197.000000\t198.000000\t199.000000\t200.000000\t201.000000\t202.000000\t203.000000\t204.000000\t205.000000\t206.000000\t207.000000\t208.000000\t209.000000\t210.000000\t211.000000\t212.000000\t213.000000\t214.000000\t215.000000\t216.000000\t217.000000\t218.000000\t219.000000\t220.000000\t221.000000\t222.000000\t223.000000\t224.000000\t225.000000\t226.000000\t227.000000\t228.000000\t229.000000\t230.000000\t231.000000\t232.000000\t233.000000\t234.000000\t235.000000\t236.000000\t237.000000\t238.000000\t239.000000\t240.000000\t241.000000\t242.000000\t243.000000\t244.000000\t245.000000\t246.000000\t247.000000\t248.000000\t249.000000\t250.000000\t251.000000\t252.000000\t253.000000\t254.000000\t255.000000\t256.000000\t257.000000\t258.000000\t259.000000\t260.000000\t261.000000\t262.000000\t263.000000\t264.000000\t265.000000\t266.000000\t267.000000\t268.000000\t269.000000\t270.000000\t271.000000\t272.000000\t273.000000\t274.000000\t275.000000\t276.000000\t277.000000\t278.000000\t279.000000\t280.000000\t281.000000\t282.000000\t283.000000\t284.000000\t285.000000\t286.000000\t287.000000\t288.000000\t289.000000\t290.000000\t291.000000\t292.000000\t293.000000\t294.000000\t295.000000\t296.000000\t297.000000\t298.000000\t299.000000\t300.000000\t301.000000\t302.000000\t303.000000\t304.000000\t305.000000\t306.000000\t307.000000\t308.000000\t309.000000\t310.000000\t311.000000\t312.000000\t313.000000\t314.000000\t315.000000\t316.000000\t317.000000\t318.000000\t319.000000\t320.000000\t321.000000\t322.000000\t323.000000\t324.000000\t325.000000\t326.000000\t327.000000\t328.000000\t329.000000\t330.000000\t331.000000\t332.000000\t333.000000\t334.000000\t335.000000\t336.000000\t337.000000\t338.000000\t339.000000\t340.000000\t341.000000\t342.000000\t343.000000\t344.000000\t345.000000\t346.000000\t347.000000\t348.000000\t349.000000\t350.000000\t351.000000\t352.000000\t353.000000\t354.000000\t355.000000\t356.000000\t357.000000\t358.000000\t359.000000\t360.000000\t361.000000\t362.000000\t363.000000\t364.000000\t365.000000\t366.000000\t367.000000\t368.000000\t369.000000\t370.000000\t371.000000\t372.000000\t373.000000\t374.000000\t375.000000\t376.000000\t377.000000\t378.000000\t379.000000\t380.000000\t381.000000\t382.000000\t383.000000\t384.000000\t385.000000\t386.000000\t387.000000\t388.000000\t389.000000\t390.000000\t391.000000\t392.000000\t393.000000\t394.000000\t395.000000\t396.000000\t397.000000\t398.000000\t399.000000\t400.000000\t401.000000\t402.000000\t403.000000\t404.000000\t405.000000\t406.000000\t407.000000\t408.000000\t409.000000\t410.000000\t411.000000\t412.000000\t413.000000\t414.000000\t415.000000\t416.000000\t417.000000\t418.000000\t419.000000\t420.000000\t421.000000\t422.000000\t423.000000\t424.000000\t425.000000\t426.000000\t427.000000\t428.000000\t429.000000\t430.000000\t431.000000\t432.000000\t433.000000\t434.000000\t435.000000\t436.000000\t437.000000\t438.000000\t439.000000\t440.000000\t441.000000\t442.000000\t443.000000\t444.000000\t445.000000\t446.000000\t447.000000\t448.000000\t449.000000\t450.000000\t451.000000\t452.000000\t453.000000\t454.000000\t455.000000\t456.000000\t457.000000\t458.000000\t459.000000\t460.000000\t461.000000\t462.000000\t463.000000\t464.000000\t465.000000\t466.000000\t467.000000\t468.000000\t469.000000\t470.000000\t471.000000\t472.000000\t473.000000\t474.000000\t475.000000\t476.000000\t477.000000\t478.000000\t479.000000\t480.000000\t481.000000\t482.000000\t483.000000\t484.000000\t485.000000\t486.000000\t487.000000\t488.000000\t489.000000\t490.000000\t491.000000\t492.000000\t493.000000\t494.000000\t495.000000\t496.000000\t497.000000\t498.000000\t499.000000\t500.000000\t501.000000\t502.000000\t503.000000\t504.000000\t505.000000\t506.000000\t507.000000\t508.000000\t509.000000\t510.000000\t511.000000\t512.000000\t513.000000\t514.000000\t515.000000\t516.000000\t517.000000\t518.000000\t519.000000\t520.000000\t521.000000\t522.000000\t523.000000\t524.000000\t525.000000\t526.000000\t527.000000\t528.000000\t529.000000\t530.000000\t531.000000\t532.000000\t533.000000\t534.000000\t535.000000\t536.000000\t537.000000\t538.000000\t539.000000\t540.000000\t541.000000\t542.000000\t543.000000\t544.000000\t545.000000\t546.000000\t547.000000\t548.000000\t549.000000\t550.000000\t551.000000\t552.000000\t553.000000\t554.000000\t555.000000\t556.000000\t557.000000\t558.000000\t559.000000\t560.000000\t561.000000\t562.000000\t563.000000\t564.000000\t565.000000\t566.000000\t567.000000\t568.000000\t569.000000\t570.000000\t571.000000\t572.000000\t573.000000\t574.000000\t575.000000\t576.000000\t577.000000\t578.000000\t579.000000\t580.000000\t581.000000\t582.000000\t583.000000\t584.000000\t585.000000\t586.000000\t587.000000\t588.000000\t589.000000\t590.000000\t591.000000\t592.000000\t593.000000\t594.000000\t595.000000\t596.000000\t597.000000\t598.000000\t599.000000\t600.000000\t601.000000\t602.000000\t603.000000\t604.000000\t605.000000\t606.000000\t607.000000\t608.000000\t609.000000\t610.000000\t611.000000\t612.000000\t613.000000\t614.000000\t615.000000\t616.000000\t617.000000\t618.000000\t619.000000\t620.000000\t621.000000\t622.000000\t623.000000\t624.000000\t625.000000\t626.000000\t627.000000\t628.000000\t629.000000\t630.000000\t631.000000\t632.000000\t633.000000\t634.000000\t635.000000\t636.000000\t637.000000\t638.000000\t639.000000\t640.000000\t641.000000\t642.000000\t643.000000\t644.000000\t645.000000\t646.000000\t647.000000\t648.000000\t649.000000\t650.000000\t651.000000\t652.000000\t653.000000\t654.000000\t655.000000" ("string T array")) -> (array=w116:dbl[][])  [unwired: 2 in]
      n36 = Index Array(array=w114, index (row)=0 ("disabled index (col)")) -> (element=w113:dbl[])  [unwired: 1 in]
      n37 = Index Array(array=w116, index (row)=0 ("disabled index (col)")) -> (element=w107:dbl[])  [unwired: 1 in]
      n38 = call <vilib>:"Derivative x(t).vi"("method"="method derivatives 3", "dt"=w125, "X"=w113) -> ("dX/dt"=w108:dbl[])  [unwired: 7 in, 1 out]
      n39 = Initialize Array(w112, 1 ("dimension size")) -> (w109:dbl[])
      n40 = call <vilib>:"Interpolate 1D.vi"("method"="method interpolation 3", "xi"=w109, "X"=w107, "Y"=w108) -> ("yi"=w123:dbl[])  [unwired: 5 in, 2 out]
      n41 = call <vilib>:"Derivative x(t).vi"("method"="method derivatives 3", "dt"=w125, "X"=w108) -> ("dX/dt"=w119:dbl[])  [unwired: 7 in, 1 out]
      n42 = Index Array(array=w123, index=0) -> (element=w111:dbl)
      n43 = call <vilib>:"Interpolate 1D.vi"("method"="method interpolation 3", "xi"=w109, "X"=w107, "Y"=w119) -> ("yi"=w121:dbl[])  [unwired: 5 in, 2 out]
      n44 = Index Array(array=w121, index=0) -> (element=w110:dbl)
    }
    frame 3 {
      w149 = 1.0 ("dt")
      # "Garberoglio et al ab initio 200 K to 2000 K"
      n45 = Spreadsheet String To Array(format string="%f", spreadsheet string="-4516.76279\n-4375.377165\n-4242.252534\n-4116.977635\n-3999.141204\n-3888.33198\n-3784.1387\n-3686.150102\n-3593.954923\n-3507.141902\n-3425.299775\n-3348.01728\n-3274.883156\n-3205.48614\n-3139.414968\n-3076.25838\n-3015.605112\n-2957.043903\n-2900.163489\n-2844.552609\n-2789.8\n-2735.568383\n-2681.816409\n-2628.576713\n-2575.881931\n-2523.764695\n-2472.257642\n-2421.393406\n-2371.204622\n-2321.723924\n-2272.983946\n-2225.017325\n-2177.856693\n-2131.534687\n-2086.083941\n-2041.537089\n-1997.926765\n-1955.285606\n-1913.646245\n-1873.041317\n-1833.503457\n-1795.0653\n-1757.75948\n-1721.618631\n-1686.668415\n-1652.890484\n-1620.249374\n-1588.709581\n-1558.235602\n-1528.791932\n-1500.34307\n-1472.853511\n-1446.287752\n-1420.610289\n-1395.78562\n-1371.77824\n-1348.552647\n-1326.073337\n-1304.304806\n-1283.211551\n-1262.758069\n-1242.908857\n-1223.62841\n-1204.881226\n-1186.631801\n-1168.844631\n-1151.484214\n-1134.515046\n-1117.901623\n-1101.608442\n-1085.6\n-1069.84649\n-1054.340895\n-1039.081895\n-1024.068169\n-1009.298397\n-994.771259\n-980.485434\n-966.439602\n-952.632442\n-939.062635\n-925.72886\n-912.629797\n-899.764125\n-887.130525\n-874.727675\n-862.554255\n-850.608946\n-838.890427\n-827.397377\n-816.128476\n-805.082404\n-794.257841\n-783.653466\n-773.267959\n-763.1\n-753.14767\n-743.40666\n-733.872061\n-724.538967\n-715.40247\n-706.457662\n-697.699634\n-689.123481\n-680.724293\n-672.497164\n-664.437185\n-656.539449\n-648.799049\n-641.211076\n-633.770623\n-626.472782\n-619.312646\n-612.285306\n-605.385856\n-598.609388\n-591.950993\n-585.405765\n-578.968795\n-572.635176\n-566.4\n-560.25897\n-554.210232\n-548.252541\n-542.384652\n-536.605323\n-530.913308\n-525.307363\n-519.786245\n-514.348708\n-508.993509\n-503.719404\n-498.525148\n-493.409497\n-488.371207\n-483.409034\n-478.521734\n-473.708061\n-468.966773\n-464.296625\n-459.696373\n-455.164772\n-450.700578\n-446.302548\n-441.969437\n-437.7\n-433.493031\n-429.347472\n-425.2623\n-421.236496\n-417.269038\n-413.358905\n-409.505076\n-405.706529\n-401.962244\n-398.271199\n-394.632373\n-391.044746\n-387.507295\n-384.019001\n-380.578841\n-377.185794\n-373.83884\n-370.536957\n-367.279125\n-364.064321\n-360.891526\n-357.759717\n-354.667874\n-351.614975\n-348.6\n-345.62203\n-342.680558\n-339.775182\n-336.905496\n-334.071098\n-331.271584\n-328.50655\n-325.775593\n-323.078308\n-320.414292\n-317.783142\n-315.184453\n-312.617823\n-310.082847\n-307.579121\n-305.106242\n-302.663807\n-300.251411\n-297.868651\n-295.515124\n-293.190425\n-290.894151\n-288.625898\n-286.385262\n-284.17184\n-281.985229\n-279.825023\n-277.690821\n-275.582217\n-273.498809\n-271.440193\n-269.405965\n-267.395721\n-265.409057\n-263.445571\n-261.504857\n-259.586514\n-257.690136\n-255.81532\n-253.961663\n-252.128761\n-250.31621\n-248.523606\n-246.750546\n-244.996627\n-243.261443\n-241.544593\n-239.845671\n-238.164275\n-236.5\n-234.852485\n-233.221534\n-231.606993\n-230.008709\n-228.426528\n-226.860295\n-225.309857\n-223.77506\n-222.255751\n-220.751774\n-219.262978\n-217.789207\n-216.330308\n-214.886127\n-213.45651\n-212.041303\n-210.640353\n-209.253506\n-207.880607\n-206.521504\n-205.176041\n-203.844066\n-202.525424\n-201.219962\n-199.927526\n-198.647961\n-197.381115\n-196.126833\n-194.884961\n-193.655346\n-192.437834\n-191.23227\n-190.038501\n-188.856374\n-187.685734\n-186.526427\n-185.3783\n-184.241199\n-183.11497\n-181.999459\n-180.894512\n-179.799976\n-178.715696\n-177.641519\n-176.577291\n-175.522858\n-174.478066\n-173.442762\n-172.416791\n-171.4\n-170.392246\n-169.393432\n-168.403472\n-167.42228\n-166.449771\n-165.485858\n-164.530455\n-163.583477\n-162.644837\n-161.71445\n-160.79223\n-159.878091\n-158.971947\n-158.073711\n-157.1833\n-156.300625\n-155.425602\n-154.558144\n-153.698165\n-152.845581\n-152.000304\n-151.162249\n-150.33133\n-149.507461\n-148.690556\n-147.880529\n-147.077295\n-146.280767\n-145.490859\n-144.707487\n-143.930562\n-143.160001\n-142.395716\n-141.637623\n-140.885634\n-140.139665\n-139.399629\n-138.66544\n-137.937013\n-137.214261\n-136.497099\n-135.785441\n-135.079201\n-134.378292\n-133.682629\n-132.992127\n-132.306699\n-131.626259\n-130.950721\n-130.28\n-129.614018\n-128.95273\n-128.2961\n-127.644092\n-126.996669\n-126.353795\n-125.715434\n-125.081549\n-124.452105\n-123.827065\n-123.206392\n-122.590051\n-121.978005\n-121.370217\n-120.766652\n-120.167273\n-119.572044\n-118.980928\n-118.39389\n-117.810893\n-117.2319\n-116.656876\n-116.085784\n-115.518587\n-114.95525\n-114.395737\n-113.84001\n-113.288034\n-112.739772\n-112.195188\n-111.654246\n-111.116909\n-110.583142\n-110.052907\n-109.526169\n-109.002891\n-108.483037\n-107.96657\n-107.453455\n-106.943655\n-106.437134\n-105.933856\n-105.433783\n-104.936881\n-104.443112\n-103.95244\n-103.464829\n-102.980243\n-102.498645\n-102.02\n-101.544274\n-101.071446\n-100.6015\n-100.134419\n-99.670186\n-99.208784\n-98.750196\n-98.294404\n-97.841393\n-97.391145\n-96.943642\n-96.498869\n-96.056807\n-95.617441\n-95.180752\n-94.746725\n-94.315341\n-93.886585\n-93.460439\n-93.036885\n-92.615908\n-92.19749\n-91.781615\n-91.368264\n-90.957421\n-90.54907\n-90.143193\n-89.739773\n-89.338793\n-88.940237\n-88.544087\n-88.150326\n-87.758937\n-87.369904\n-86.983209\n-86.598835\n-86.216765\n-85.836983\n-85.459472\n-85.084213\n-84.711191\n-84.340389\n-83.971789\n-83.605374\n-83.241128\n-82.879033\n-82.519073\n-82.16123\n-81.805488\n-81.451829") -> (array=w135:dbl[][])  [unwired: 2 in]
      n46 = Spreadsheet String To Array(format string="%f", spreadsheet string="230\n231\n232\n233\n234\n235\n236\n237\n238\n239\n240\n241\n242\n243\n244\n245\n246\n247\n248\n249\n250\n251\n252\n253\n254\n255\n256\n257\n258\n259\n260\n261\n262\n263\n264\n265\n266\n267\n268\n269\n270\n271\n272\n273\n274\n275\n276\n277\n278\n279\n280\n281\n282\n283\n284\n285\n286\n287\n288\n289\n290\n291\n292\n293\n294\n295\n296\n297\n298\n299\n300\n301\n302\n303\n304\n305\n306\n307\n308\n309\n310\n311\n312\n313\n314\n315\n316\n317\n318\n319\n320\n321\n322\n323\n324\n325\n326\n327\n328\n329\n330\n331\n332\n333\n334\n335\n336\n337\n338\n339\n340\n341\n342\n343\n344\n345\n346\n347\n348\n349\n350\n351\n352\n353\n354\n355\n356\n357\n358\n359\n360\n361\n362\n363\n364\n365\n366\n367\n368\n369\n370\n371\n372\n373\n374\n375\n376\n377\n378\n379\n...") -> (array=w138:dbl[][])  [unwired: 2 in]
      n47 = Index Array(array=w135, index (col)=0 ("disabled index (col)")) -> (element=w133:dbl[])  [unwired: 1 in]
      n48 = Index Array(array=w138, index (col)=0 ("disabled index (col)")) -> (element=w128:dbl[])  [unwired: 1 in]
      n49 = call <vilib>:"Derivative x(t).vi"("method"="method derivatives 4", "dt"=w149, "X"=w133) -> ("dX/dt"=w142:dbl[])  [unwired: 7 in, 1 out]
      n50 = Initialize Array(w131, 1 ("dimension size")) -> (w141:dbl[])
      n51 = call <vilib>:"Interpolate 1D.vi"("method"="method interpolation 4", "xi"=w141, "X"=w128, "Y"=w142) -> ("yi"=w147:dbl[])  [unwired: 5 in, 2 out]
      n52 = call <vilib>:"Derivative x(t).vi"("method"="method derivatives 4", "dt"=w149, "X"=w142) -> ("dX/dt"=w143:dbl[])  [unwired: 7 in, 1 out]
      n53 = Index Array(array=w147, index=0) -> (element=w129:dbl)
      n54 = call <vilib>:"Interpolate 1D.vi"("method"="method interpolation 4", "xi"=w141, "X"=w128, "Y"=w143) -> ("yi"=w145:dbl[])  [unwired: 5 in, 2 out]
      n55 = Index Array(array=w145, index=0) -> (element=w130:dbl)
    }
    frame 4 {
      # "cm^3/mol"
      # "Square well fitted from IAPWS data"
      n56 = formula code="dB=((b*c)/(T*T))*exp(c/T);\nd2B= -(((b*c*c)/(T*T*T*T))+((2*b*c)/(T*T*T)))*exp(c/T);"("T"=w151, "a"=-27.78, "b"=5.55063, "c"=1609.145) -> ("dB"=w153:dbl, "d2B"=w152:dbl)
    }
  }
  n57 = case shown="0, Default" "B source ref dry air" {
    tunnel: [w170 w183] -> w26
    tunnel: [w169 w182] -> w24
    tunnel: "Temperature (K)" -> [w177 w181]
    frame 0, Default {
      w179 = 1.0 ("dt")
      # "B(T) dry air Lemmon EOS imp. by REFPPROP 200 K - 700 K"
      n58 = Spreadsheet String To Array(format string="%f", spreadsheet string="-39.27226\n-38.76521\n-38.2643\n-37.76942\n-37.28047\n-36.79734\n-36.31992\n-35.84813\n-35.38185\n-34.92101\n-34.4655\n-34.01523\n-33.57012\n-33.13008\n-32.69502\n-32.26487\n-31.83953\n-31.41894\n-31.00301\n-30.59167\n-30.18485\n-29.78246\n-29.38445\n-28.99075\n-28.60127\n-28.21597\n-27.83476\n-27.4576\n-27.08441\n-26.71514\n-26.34972\n-25.9881\n-25.63022\n-25.27602\n-24.92545\n-24.57846\n-24.23498\n-23.89498\n-23.55839\n-23.22517\n-22.89527\n-22.56864\n-22.24523\n-21.925\n-21.60791\n-21.2939\n-20.98294\n-20.67498\n-20.36998\n-20.0679\n-19.76869\n-19.47233\n-19.17876\n-18.88795\n-18.59987\n-18.31448\n-18.03173\n-17.7516\n-17.47405\n-17.19905\n-16.92655\n-16.65654\n-16.38897\n-16.12382\n-15.86105\n-15.60063\n-15.34254\n-15.08673\n-14.83319\n-14.58188\n-14.33278\n-14.08585\n-13.84108\n-13.59843\n-13.35787\n-13.11939\n-12.88295\n-12.64853\n-12.41611\n-12.18566\n-11.95715\n-11.73057\n-11.50588\n-11.28308\n-11.06213\n-10.84301\n-10.6257\n-10.41018\n-10.19643\n-9.984431\n-9.774155\n-9.565587\n-9.358706\n-9.153492\n-8.949926\n-8.74799\n-8.547665\n-8.348932\n-8.151774\n-7.956172\n-7.76211\n-7.569569\n-7.378533\n-7.188985\n-7.000908\n-6.814287\n-6.629105\n-6.445346\n-6.262995\n-6.082036\n-5.902455\n-5.724236\n-5.547365\n-5.371827\n-5.197607\n-5.024693\n-4.85307\n-4.682724\n-4.513641\n-4.34581\n-4.179215\n-4.013845\n-3.849686\n-3.686727\n-3.524954\n-3.364355\n-3.204919\n-3.046633\n-2.889486\n-2.733466\n-2.578561\n-2.424761\n-2.272054\n-2.120429\n-1.969875\n-1.820382\n-1.671939\n-1.524536\n-1.378162\n-1.232807\n-1.088461\n-0.9451149\n-0.8027581\n-0.6613813\n-0.5209748\n-0.3815294\n-0.2430356\n-0.1054845\n0.03113316\n0.1668262\n0.3016034\n0.4354735\n0.5684451\n0.7005267\n0.8317267\n0.9620533\n1.091515\n1.220119\n1.347874\n1.474788\n1.600869\n1.726123\n1.85056\n1.974185\n2.097008\n2.219034\n2.340272\n2.460728\n2.58041\n2.699324\n2.817478\n2.934877\n3.05153\n3.167442\n3.282621\n3.397072\n3.510802\n3.623817\n3.736124\n3.84773\n3.958639\n4.068858\n4.178394\n4.287251\n4.395436\n4.502955\n4.609814\n4.716018\n4.821572\n4.926482\n5.030754\n5.134394\n5.237406\n5.339795\n5.441568\n5.542728\n5.643282\n5.743235\n5.84259\n5.941354\n6.039532\n6.137127\n6.234145\n6.330591\n6.426469\n6.521785\n6.616541\n6.710744\n6.804397\n6.897506\n6.990074\n7.082105\n7.173605\n7.264577\n7.355026\n7.444955\n7.53437\n7.623273\n7.71167\n7.799563\n7.886957\n7.973857\n8.060265\n8.146186\n8.231623\n8.31658\n8.401062\n8.48507\n8.568611\n8.651686\n8.734299\n8.816455\n8.898156\n8.979406\n9.060209\n9.140567\n9.220484\n9.299964\n9.37901\n9.457625\n9.535812\n9.613575\n9.690917\n9.76784\n9.844348\n9.920445\n9.996132\n10.07141\n10.14629\n10.22077\n10.29485\n10.36854\n10.44184\n10.51475\n10.58727\n10.65941\n10.73117\n10.80255\n10.87356\n10.9442\n11.01446\n11.08437\n11.1539\n11.22308\n11.2919\n11.36036\n11.42847\n11.49622\n11.56363\n11.63069\n11.69741\n11.76379\n11.82983\n11.89553\n11.96089\n12.02593\n12.09063\n12.15501\n12.21907\n12.2828\n12.34621\n12.4093\n12.47207\n12.53454\n12.59669\n12.65853\n12.72006\n12.78128\n12.84221\n12.90283\n12.96315\n13.02318\n13.08291\n13.14234\n13.20149\n13.26034\n13.31891\n13.37719\n13.43519\n13.4929\n13.55034\n13.6075\n13.66438\n13.72099\n13.77732\n13.83338\n13.88918\n13.94471\n13.99997\n14.05496\n14.1097\n14.16417\n14.21839\n14.27235\n14.32605\n14.3795\n14.43269\n14.48564\n14.53834\n14.59078\n14.64299\n14.69495\n14.74666\n14.79814\n14.84937\n14.90037\n14.95113\n15.00165\n15.05194\n15.102\n15.15183\n15.20143\n15.2508\n15.29994\n15.34886\n15.39756\n15.44603\n15.49428\n15.54231\n15.59012\n15.63772\n15.6851\n15.73227\n15.77922\n15.82596\n15.87249\n15.91881\n15.96493\n16.01083\n16.05654\n16.10203\n16.14733\n16.19242\n16.23731\n16.282\n16.3265\n16.3708\n16.4149\n16.4588\n16.50252\n16.54604\n16.58937\n16.63251\n16.67546\n16.71822\n16.7608\n16.80319\n16.8454\n16.88742\n16.92926\n16.97092\n17.01239\n17.05369\n17.09481\n17.13576\n17.17652\n17.21712\n17.25753\n17.29778\n17.33785\n17.37775\n17.41748\n17.45704\n17.49644\n17.53566\n17.57472\n17.61362\n17.65235\n17.69091\n17.72932\n17.76756\n17.80564\n17.84356\n17.88132\n17.91892\n17.95637\n17.99366\n18.03079\n18.06777\n18.1046\n18.14127\n18.17779\n18.21416\n18.25038\n18.28645\n18.32237\n18.35814\n18.39377\n18.42925\n18.46458\n18.49977\n18.53481\n18.56971\n18.60447\n18.63909\n18.67357\n18.7079\n18.7421\n18.77615\n18.81007\n18.84386\n18.8775\n18.91101\n18.94439\n18.97763\n19.01074\n19.04371\n19.07656\n19.10927\n19.14185\n19.1743\n19.20662\n19.23881\n19.27087\n19.30281\n19.33462\n19.36631\n19.39786\n19.4293\n19.46061\n19.4918\n19.52286\n19.5538\n19.58462\n19.61532\n19.6459\n19.67636\n19.7067\n19.73692\n19.76702\n19.79701\n19.82688\n19.85664\n19.88627\n19.9158\n19.94521\n19.9745\n20.00369\n20.03276\n20.06172\n20.09056\n20.1193\n20.14792\n20.17644\n20.20485\n20.23315\n20.26134\n20.28942\n20.3174\n20.34526\n20.37303\n20.40069\n20.42824\n20.45569\n20.48303\n20.51027\n20.53741\n20.56445\n20.59138\n20.61822\n20.64495\n20.67158\n20.69811\n20.72455\n20.75088\n20.77712\n20.80325\n20.82929\n20.85524\n20.88108\n20.90684\n20.93249\n20.95805\n20.98352\n21.00889\n21.03416\n21.05935\n21.08444\n21.10944\n21.13435\n21.15916") -> (array=w162:dbl[][])  [unwired: 2 in]
      n59 = Spreadsheet String To Array(format string="%f", spreadsheet string="200\n201\n202\n203\n204\n205\n206\n207\n208\n209\n210\n211\n212\n213\n214\n215\n216\n217\n218\n219\n220\n221\n222\n223\n224\n225\n226\n227\n228\n229\n230\n231\n232\n233\n234\n235\n236\n237\n238\n239\n240\n241\n242\n243\n244\n245\n246\n247\n248\n249\n250\n251\n252\n253\n254\n255\n256\n257\n258\n259\n260\n261\n262\n263\n264\n265\n266\n267\n268\n269\n270\n271\n272\n273\n274\n275\n276\n277\n278\n279\n280\n281\n282\n283\n284\n285\n286\n287\n288\n289\n290\n291\n292\n293\n294\n295\n296\n297\n298\n299\n300\n301\n302\n303\n304\n305\n306\n307\n308\n309\n310\n311\n312\n313\n314\n315\n316\n317\n318\n319\n320\n321\n322\n323\n324\n325\n326\n327\n328\n329\n330\n331\n332\n333\n334\n335\n336\n337\n338\n339\n340\n341\n342\n343\n344\n345\n346\n347\n348\n349\n...") -> (array=w165:dbl[][])  [unwired: 2 in]
      n60 = Index Array(array=w162, index (col)=0 ("disabled index (col)")) -> (element=w158:dbl[])  [unwired: 1 in]
      n61 = Index Array(array=w165, index (col)=0 ("disabled index (col)")) -> (element=w157:dbl[])  [unwired: 1 in]
      n62 = call <vilib>:"Derivative x(t).vi"("method"="method derivatives", "dt"=w179, "X"=w158) -> ("dX/dt"=w171:dbl[])  [unwired: 7 in, 1 out]
      n63 = Initialize Array(w177, 1 ("dimension size")) -> (w168:dbl[])
      n64 = call <vilib>:"Interpolate 1D.vi"("method"="method interpolation", "xi"=w168, "X"=w157, "Y"=w171) -> ("yi"=w176:dbl[])  [unwired: 5 in, 2 out]
      n65 = call <vilib>:"Derivative x(t).vi"("method"="method derivatives", "dt"=w179, "X"=w171) -> ("dX/dt"=w172:dbl[])  [unwired: 7 in, 1 out]
      n66 = Index Array(array=w176, index=0) -> (element=w170:dbl)
      n67 = call <vilib>:"Interpolate 1D.vi"("method"="method interpolation", "xi"=w168, "X"=w157, "Y"=w172) -> ("yi"=w174:dbl[])  [unwired: 5 in, 2 out]
      n68 = Index Array(array=w174, index=0) -> (element=w169:dbl)
    }
    frame 1 {
      # "B(T) dry air Zuckerwar square well fit to data and correlations 230 K - 650 K"
      # "cm^3/mol"
      n69 = formula code="dB=((b*c)/(T*T))*exp(c/T);\nd2B= -(((b*c*c)/(T*T*T*T))+((2*b*c)/(T*T*T)))*exp(c/T);"("T"=w181, "a"=152.2 ("input variable"), "b"=111.3 ("input variable"), "c"=108.1 ("input variable")) -> ("dB"=w183:dbl, "d2B"=w182:dbl)
    }
  }
  n70 = Multiply(x=w23, y=w24) -> (x*y=w17:dbl)
  "d^2Bair/dT^2" <- w17
  n71 = Multiply(x=w25, y=w22) -> (x*y=w15:dbl)
  "dBwater/dT" <- w15
  n72 = Multiply(x=w22, y=w21) -> (x*y=w16:dbl)
  "d^2Bwater/dT^2" <- w16
  n73 = Multiply(x=w26, y=w23) -> (x*y=w20:dbl)
  "dBair/dT" <- w20
  n74 = Multiply(x=w10, y=w12) -> (x*y=w8:dbl)
  "dBair-water/dT" <- w8
  n75 = Multiply(x=w12, y=w11) -> (x*y=w5:dbl)
  "d^2Bair-water/dT^2" <- w5
  n76 = global write "SOS_Global_2022.vi" "d^2Ba(T)/dT^2"(w17) -> ()
  n77 = global write "SOS_Global_2022.vi" "dBa(T)/dT"(w20) -> ()
  n78 = global write "SOS_Global_2022.vi" "d^2Bw(T)/dT^2"(w16) -> ()
  n79 = global write "SOS_Global_2022.vi" "dBw(T)/dT"(w15) -> ()
  n80 = Square(x="Temperature (K)") -> (x^2=w6:dbl)
  n81 = Multiply(x=w20, y="Temperature (K)") -> (x*y=→"T*dBair/dT":dbl)
  n82 = Multiply(x=w15, y="Temperature (K)") -> (x*y=→"T*dBwater/dT":dbl)
  n83 = Multiply(x="Temperature (K)", y=w8) -> (x*y=→"T*dBair-water/dT":dbl)
  n84 = Multiply(x=w17, y=w6) -> (x*y=→"T^2*d^2Bair/dT^2":dbl)
  n85 = Multiply(x=w16, y=w6) -> (x*y=→"T^2*d^2Bwater/dT^2":dbl)
  n86 = Multiply(x=w6, y=w5) -> (x*y=→"T^2*d^2Bair-water/dT^2":dbl)
